vi "scale display.vi"(2 "Data Display":T1 {"average data rate (Hz)" format="%.2f"; "Min Range" format="%.3f"; "Max Range" format="%.3f"; "Mean (Volts)" format="%.5f"; "Mean (scaled)" format="%.2f"}, 3 "Index":u32) -> ()   [LabVIEW 2010]
uses:
  calibrator graph.ctl
  <vilib>/Analysis/1siggen.llb/Ramp Pattern by Samples.vi
  global scale array.vi
  <vilib>/Analysis/NI_AALBase.lvlib
panel:
  in  "OK Button":bool
  out "Calibration Graph":cluster{"Ramp Pattern":dbl[], sgl[]}(graph)
  # "The potential sensor output given the voltage range of the selected port. \nThe sensor may not be able to use the entire voltage range."
  # "V"
  # "V"
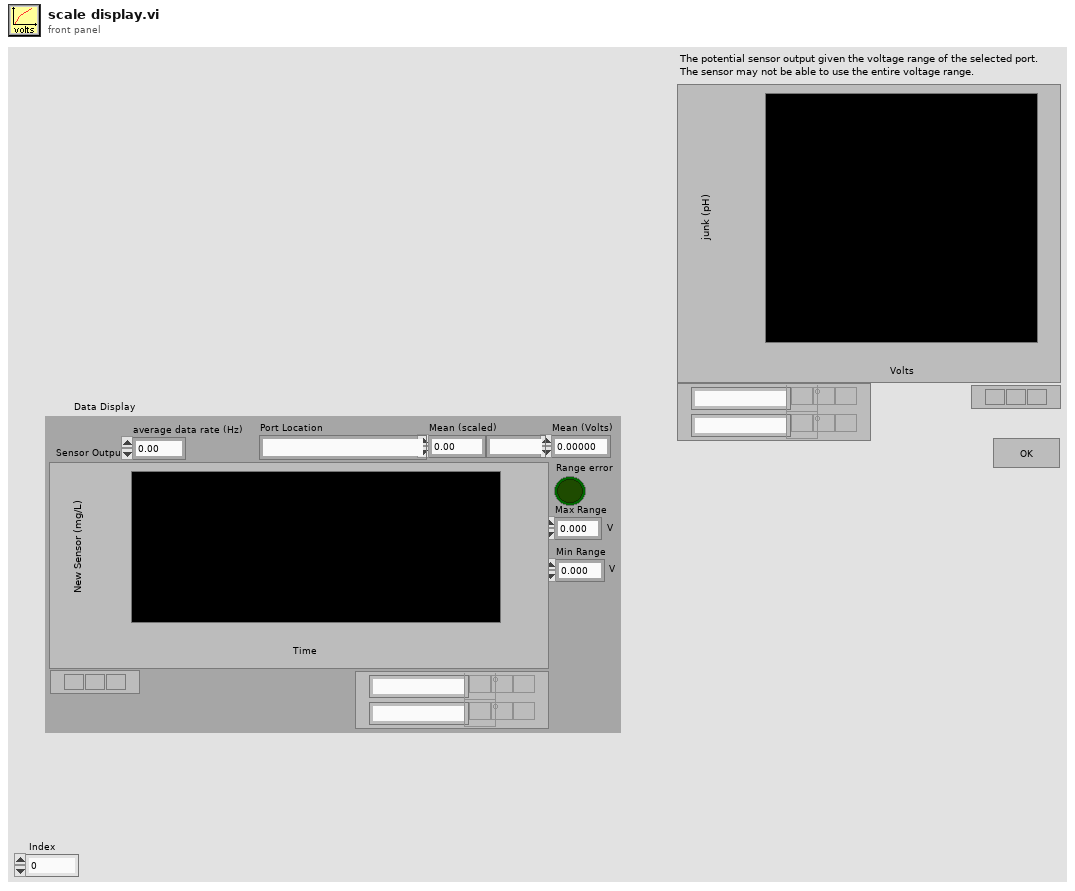
[diagram p1: front panel]
types:
  T1 = typedef "calibrator graph.ctl" = cluster{"Range error":bool, "Mean (scaled)":dbl, "Mean (Volts)":dbl, "Max Range":dbl, "Min Range":dbl, "units":string, "Sensor Output":cluster{dbl[], dbl[]}[], "Port Location":string, "average data rate (Hz)":dbl}
  T2 = typedef "calib array.ctl" = T3[]
  T3 = typedef "conversion.ctl" = cluster{"conversion matrix":sgl[][], "units":string, "name":string, "scale type":T4, "offset (volts)":dbl, "second channel":i8, "correspondence table":T5, "offset (physical units)":dbl, "pH scale":T6, "D.O.":T7}
  T4 = typedef "scale type.ctl" = enum16{"Volts", "Polynomial", "Correspondence Table", "pH", "Dissolved Oxygen", "Quadratic"}
  T5 = typedef "correspondence table.ctl" = cluster{"physical units":dbl, "volts":dbl}[]
  T6 = typedef "pH scale.ctl" = cluster{"Buffers":cluster{"Buffer":dbl, "Calibrated":bool, "V/T":dbl}[], "Temperature":dbl}
  T7 = typedef "DO scale.ctl" = cluster{"Temperature":dbl, "K":dbl, "barometric pressure":dbl}
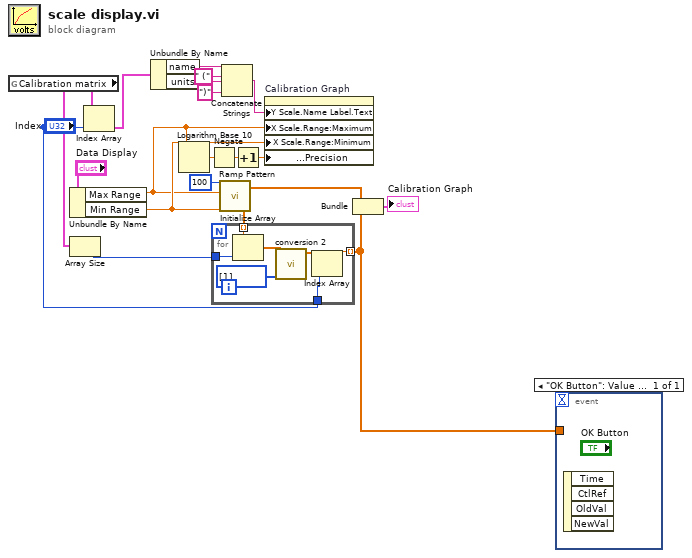
[diagram p0: block diagram]
diagram:
  n1 = global read "global scale array.vi" "Calibration matrix"() -> (w18:T2)
  n2 = Unbundle By Name("Data Display") -> ("Max Range"=w5:dbl, "Min Range"=w7:dbl)
  n3 = Array Size(array=w18) -> (size(s)=w1:i32)
  n4 = Index Array(array=w18, index="Index") -> (element=w13:T3)
  n5 = Unbundle By Name(w13) -> ("name"=w12:string, "units"=w10:string)
  n6 = Logarithm Base 10(1:w5) -> (0:w6:dbl)
  n7 = Negate(x=w6) -> (-x=w4:dbl)
  n8 = call-poly <vilib>:"Ramp Pattern.vi"("start"=w7, "end"=w5, "samples"=100) -> ("Ramp Pattern"=w15:dbl[])  [unwired: 7 in, 1 out]
  n9 = for {
    tunnel: w15 -> [w24] mode=indexing
    tunnel: [w25] -> w2 mode=indexing
    tunnel: w1 -> [w23]
    tunnel: "Index" -> [w21]
    n10 = Initialize Array(w24, w23) -> (w22:dbl[])
    n11 = call "conversion 2.vi"("Channel Indices"=u8[] [1], "voltage data"=w22) -> ("calibrated data"=w26:sgl[])  [unwired: 8 in, 1 out]
    n12 = Index Array(array=w26, index=w21) -> (element=w25:sgl)
  }
  n13 = Concatenate Strings(w12, " (" ("Substring"), w10, ")" ("Substring")) -> (w8:string)
  n14 = Increment(x=w4) -> (x+1=w3:dbl)
  n15 = property on="Calibration Graph" class="XYGraph (strict)"("Y Scale.Name Label.Text"=w8, "X Scale.Range:Maximum"=w5, "X Scale.Range:Minimum"=w7, "X Scale.Format & Precision:Precision"=w3) -> ()  [unwired: 2 in, 2 out]
  n16 = Bundle("Ramp Pattern"=w15, w2) -> (→"Calibration Graph":cluster{"Ramp Pattern":dbl[], sgl[]})  [unwired: 1 in]
  n17 = event shown="[0] \"OK Button\": Value Change" {
    selector: _ -> [_]
    dyn-events: _ -> [_]
    timeout: _ -> [_]
    tunnel: w2 -> [_]
    event "OK Button": Value Change {
      n18 = event-data() -> ()  [unwired: 1 in, 4 out]
    }
  }
